vi "Step Prompt.vi"(0 "VISA resource name":refnum<visa-resource-name>, 5 "Prompt ( )":string=" ", 11 "error in (no error)":errorcluster) -> (4 "VISA resource name out":refnum<visa-resource-name>, 15 "error out":errorcluster)   [LabVIEW 2020, in "eec 6700.lvlib"]
doc: "Sets the <B>Step Prompt</B> in the active step of the current Memory location (Use \"Configure Memory.vi\" to select the desired memory)\n\nNiote : Only for Program mode. Make sure the instrument is set to the program mode and then the prefered step for prompt is set as the active step.\n\nPrompt is an Alphanumeric parameter.\n\nThe prompt parameter setting configures a message unique to a particular step. The message will be shown on the LCD graphic display prior to the test beginning for that particular step test routine. At this point the test routine will be interrupted and the operator must press the text/reset key to begin the test sequence."
uses:
  <instrlib>/eec 6700/eec 6700.lvlib
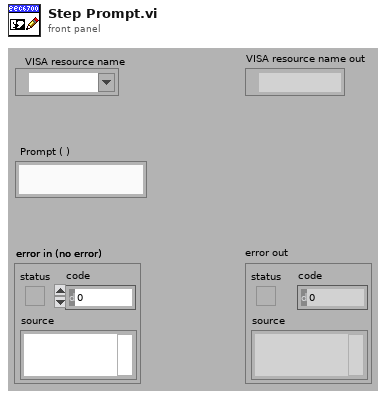
[diagram p1: front panel]
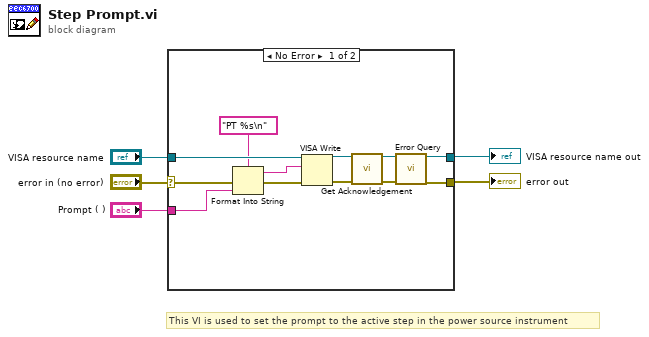
[diagram p0: block diagram]
diagram:
  # "This VI is used to set the prompt to the active step in the power source instrument"
  n1 = case shown="No Error" "error in (no error)" {
    selector: "error in (no error)" -> [w11 w19]
    tunnel: "VISA resource name" -> [w17 w18]
    tunnel: [w13 w18] -> w4
    tunnel: [w12 w19] -> w3
    tunnel: "Prompt ( )" -> [w16 _]
    frame No Error {
      n2 = Format Into String(format string="PT %s\n" ("Command"), error in=w11, w16) -> (resulting string=w15:string, error out=w10:errorcluster)  [unwired: 1 in]
      n3 = VISA Write(VISA resource name=w17, write buffer=w15, error in (no error)=w10) -> (VISA resource name out=w6:refnum<visa-resource-name>, error out=w7:errorcluster)  [unwired: 1 out]
      n4 = call <instrlib>:"Get Acknowledgement.vi"("VISA resource name"=w6, "error in (no error)"=w7) -> ("VISA resource name out"=w9:refnum<visa-resource-name>, "error out"=w8:errorcluster)  [unwired: 12 in]
      n5 = call <instrlib>:"Error Query.vi"("VISA resource name"=w9, "error in (no error)"=w8) -> ("VISA resource name out"=w13:refnum<visa-resource-name>, "error out"=w12:errorcluster)  [unwired: 10 in, 2 out]
    }
    frame Error {
    }
  }
  "error out" <- w3
  "VISA resource name out" <- w4
